vi "imaqrio_CloseImpl.vi"(4 "error in (no error)":errorcluster, 6 "Options (Abort, Close)":enum16{"Abort, Close", "Close"}(ring), 7 "HW Exec Ref":refnum<visa-resource-name>) -> (0 "error out":errorcluster)   [LabVIEW 2017]
doc: "This sub VI at the very least closes open references and possibly aborts the VI."
panel:
  in  "HW Exec Ref Cluster":T1
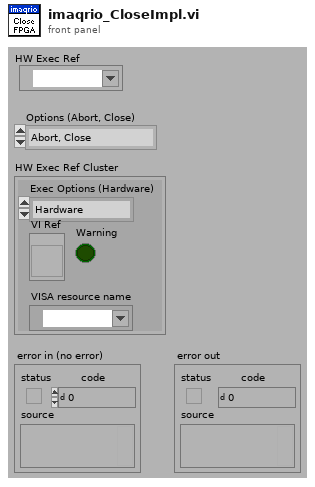
[diagram p1: front panel]
types:
  T1 = cluster{"Exec Options (Hardware)":enum16{"Hardware", "Simulation"}, "VI Ref":refnum<vi>, "VISA resource name":refnum<visa-resource-name>, "Warning":bool}
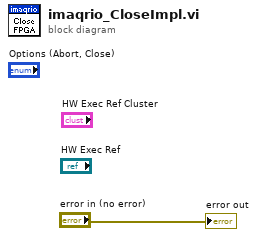
[diagram p0: block diagram]
diagram:
  "error out" <- "error in (no error)"
